vi "test_cavity_model.vi"() -> ()   [LabVIEW 2013]
uses:
  <vilib>/measure/NI_MABase.lvlib
panel:
  out "Waveform Graph 4":dbl[](graph)
  out "Waveform Graph 3":dbl[](graph)
  out "Waveform Graph 2":dbl[](graph)
  out "Waveform Graph":dbl[](graph)
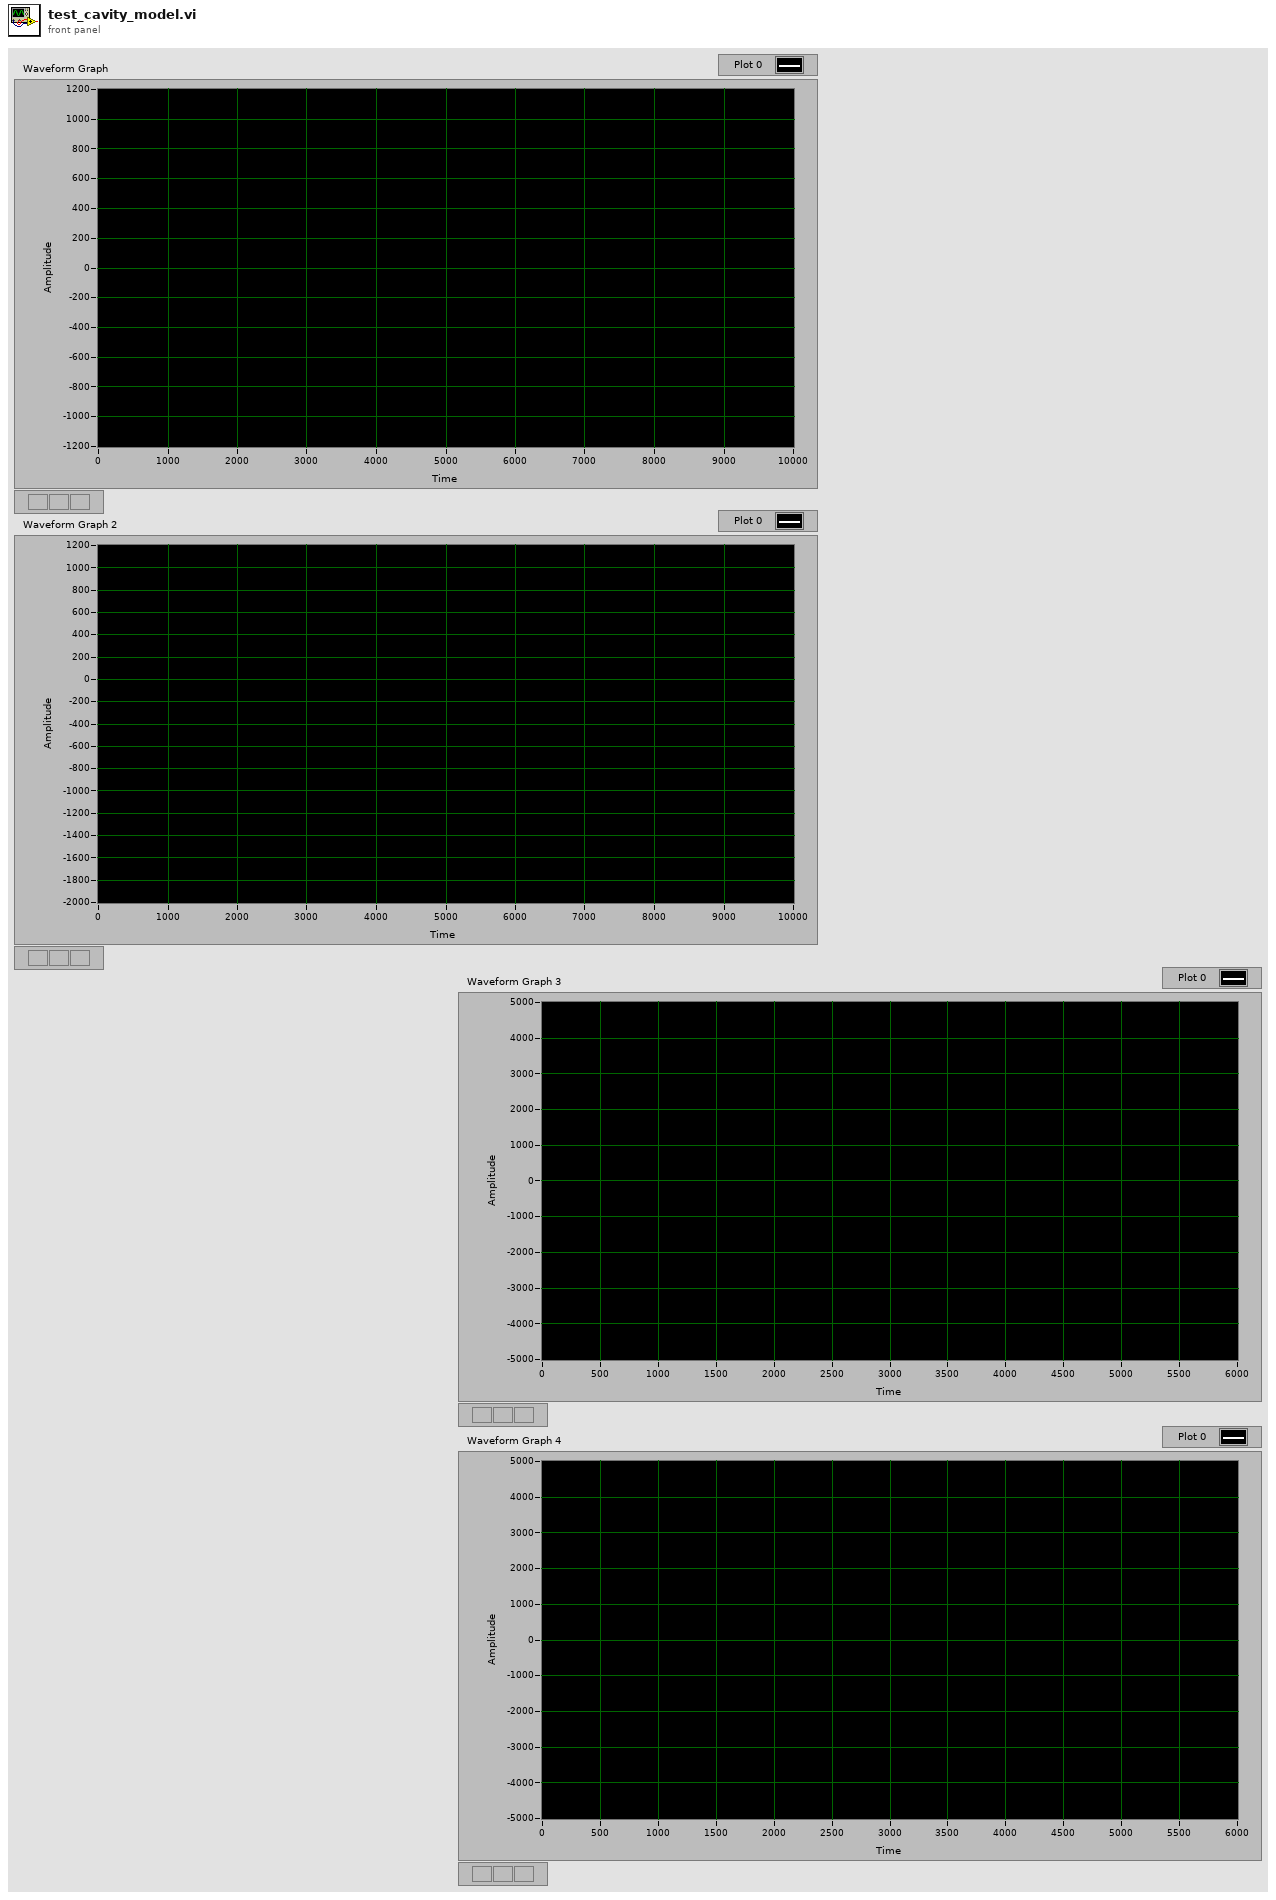
[diagram p1: front panel]
types:
  T1 = cluster{"frequency":dbl, "amplitude":dbl, "phase":dbl}[]
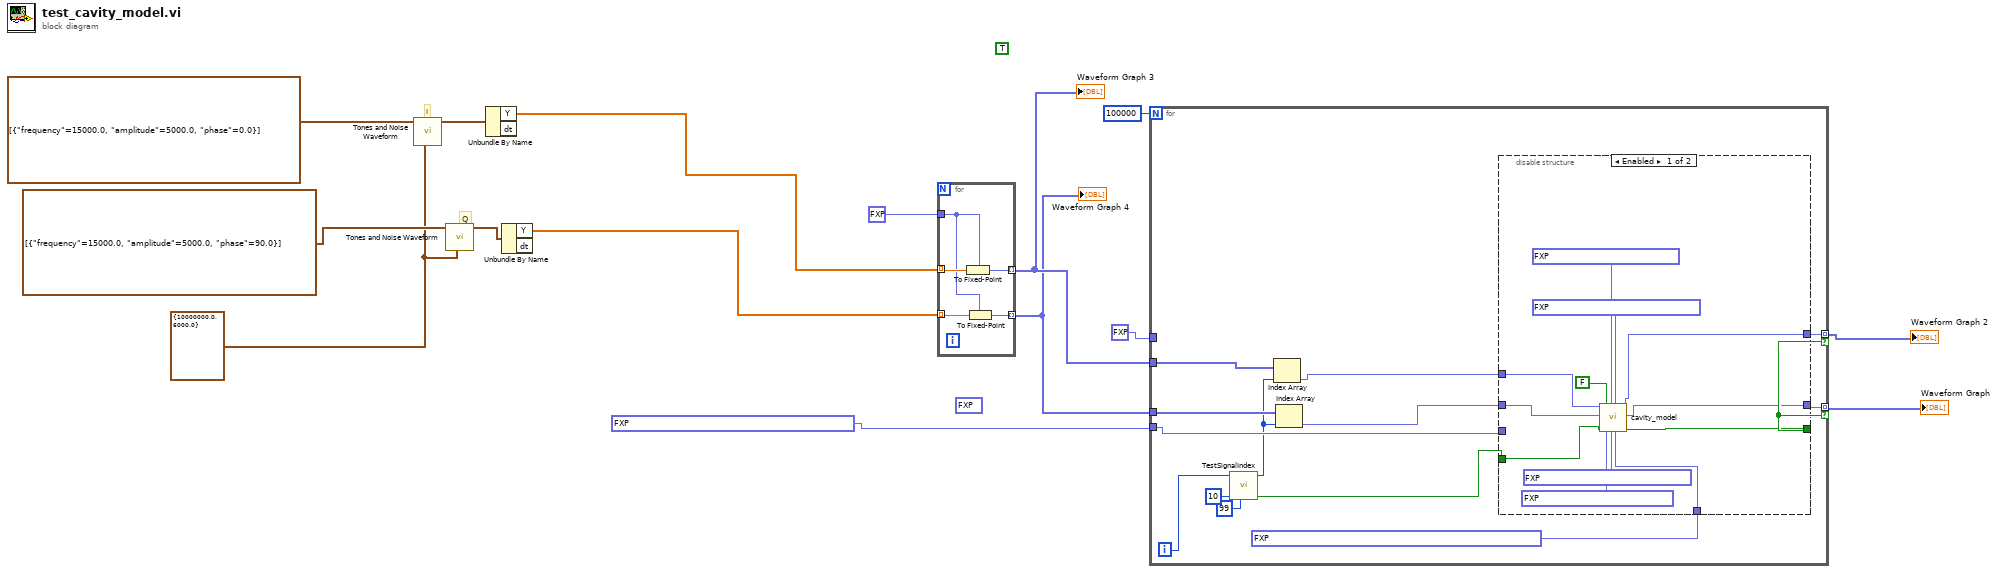
[diagram p0: block diagram]
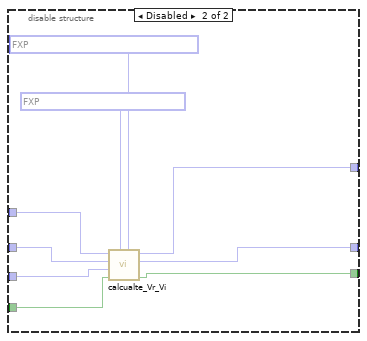
[diagram p2: hidden frame]
diagram:
  (unwired) TRUE
  w7 = cluster{"Fs":dbl, "#s":dbl} {"Fs"=10000000.0, "#s"=6000.0} ("sampling info")
  (unwired) fxp<+/-,16,14> 4000.0 ("Ii")
  # "Q"
  # "I"
  n1 = call <vilib>:"Tones and Noise Waveform.vi"("sampling info"=w7, "tones"=T1 [{"frequency"=15000.0, "amplitude"=5000.0, "phase"=0.0}]) -> ("signal out"=w9:waveform(dbl))  [unwired: 8 in, 1 out]
  n2 = call <vilib>:"Tones and Noise Waveform.vi"("sampling info"=w7, "tones"=T1 [{"frequency"=15000.0, "amplitude"=5000.0, "phase"=90.0}]) -> ("signal out"=w6:waveform(dbl))  [unwired: 8 in, 1 out]
  n3 = Unbundle By Name(w9) -> ("Y"=w5:dbl[])  [unwired: 1 out]
  n4 = Unbundle By Name(w6) -> ("Y"=w4:dbl[])  [unwired: 1 out]
  n5 = for {
    tunnel: w4 -> [w20] mode=indexing
    tunnel: fxp<+/-,16,14> 0.0 ("fixed-point type") -> [w16]
    tunnel: [w19] -> w1 mode=indexing
    tunnel: w5 -> [w17] mode=indexing
    tunnel: [w18] -> w2 mode=indexing
    n6 = To Fixed-Point(fixed-point type=w16, number=w17) -> (fixed-point=w18:fxp<+/-,16,14>)
    n7 = To Fixed-Point(fixed-point type=w16, number=w20) -> (fixed-point=w19:fxp<+/-,16,14>)
  }
  "Waveform Graph 3" <- w2
  "Waveform Graph 4" <- w1
  n8 = for {
    N: 100000 -> [_]
    tunnel: [w34] -> w14 mode=indexing if=w21
    tunnel: fxp<+/-,48,0> 5.000000058430487e-08 ("dw*dt") -> [w33]
    tunnel: fxp<+/-,16,14> 0.0 ("Ii") -> [_]
    tunnel: [w32] -> w13 mode=indexing if=w21
    tunnel: w2 -> [w28]
    tunnel: w1 -> [w27]
    i -> [w25]
    n9 = call "TestSignalIndex.vi"("initial delay"=99, "cycles per sample"=10, "index"=w25) -> ("valid out"=w29:bool, "array index"=w26:i32)  [unwired: 7 in]
    n10 = Index Array(array=w28, index=w26) -> (element=w24:fxp<+/-,16,14>)
    n11 = Index Array(array=w27, index=w26) -> (element=w23:fxp<+/-,16,14>)
    n12 = disable-structure shown="Enabled" {
      disable-tunnel: w24 -> [w46 w55]
      disable-tunnel: w29 -> [w45 w53]
      disable-tunnel: [w43 w48] -> w34
      disable-tunnel: [w44 w47] -> w21
      disable-tunnel: w33 -> [_ w54]
      disable-tunnel: w23 -> [w42 w52]
      disable-tunnel: [w41 w49] -> w32
      disable-tunnel: fxp<+/-,32,-32> -5.479427675481041e-14 ("C5") -> [w36 _]
      frame Enabled {
        n13 = call "cavity_model.vi"("Ir"=w46, "Ii"=w42, "input valid"=w45, "reset"=FALSE, "C3"=fxp<+/-,32,3> -2.180195599794388, "C1"=fxp<+/-,32,3> 0.9986428320407867, "C4"=fxp<+/-,32,2> 0.999985234811902, "C2"=fxp<+/-,32,3> 0.002117181196808815, "C5"=w36) -> ("Vr"=w41:fxp<+/-,16,14>, "Vi"=w43:fxp<+/-,16,14>, "output valid"=w44:bool)  [unwired: 8 in]
      }
      frame Disabled {
        n14 = call "calcualte_Vr_Vi.vi"("C2"=fxp<+/-,32,3> 0.002117181196808815, "C1"=fxp<+/-,32,3> 0.9986428320407867, "input valid"=w53, "dw*dt"=w54, "Ii"=w52, "Ir"=w55) -> ("output valid"=w47:bool, "Vi"=w48:fxp<+/-,48,16>, "Vr"=w49:fxp<+/-,48,16>)  [unwired: 3 in]
      }
    }
  }
  "Waveform Graph" <- w14
  "Waveform Graph 2" <- w13
